vi "Get driving mode to excecute.vi"() -> (2 "Drive Mode":T1)   [LabVIEW 2018]
uses:
  Drive mode.ctl
panel:
  # "Choose which mode to excecute"
  # "IDK HOw this is going to work exactly"
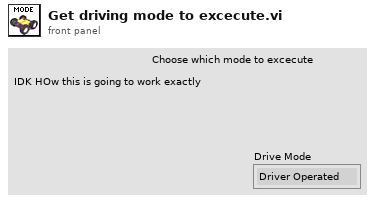
[diagram p1: front panel]
types:
  T1 = typedef "Drive mode.ctl" = enum16{"Driver Operated", "Drive Autonomously"}
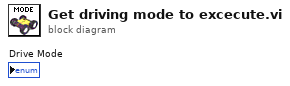
[diagram p0: block diagram]
diagram:
